vi "Set Output State.vi"(7 "Output Channel":T2, 8 "error in (no error)":errorcluster, 10 "Output State":T1=enum."Enabled", 11 "VISA resource name":refnum<visa-resource-name>) -> (0 "error out":errorcluster, 3 "VISA Refnum out":refnum<visa-resource-name>)   [LabVIEW 2016, in "RP100.lvclass"]
uses:
  RP100.lvclass
  Typedefs/Output Channel--Enum.ctl
  Typedefs/Output State--Enum.ctl
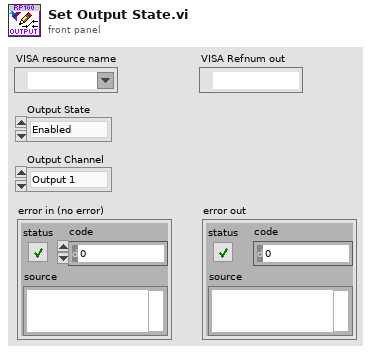
[diagram p1: front panel]
types:
  T1 = typedef "RP100.lvclass/Output State--Enum.ctl" = enum16{"Shorted", "Enabled"}
  T2 = typedef "RP100.lvclass/Output Channel--Enum.ctl" = enum16{"Output 1", "Output 2"}
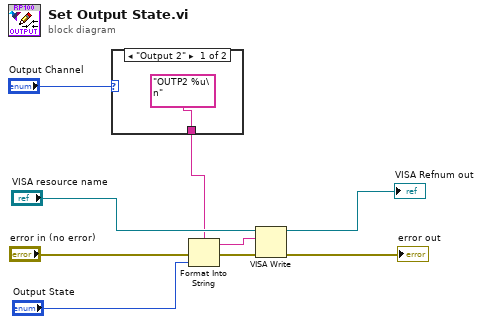
[diagram p0: block diagram]
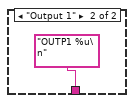
[diagram p2: hidden frame]
diagram:
  n1 = case shown="\"Output 2\"" "Output Channel" {
    tunnel: ["OUTP2 %u\n" ("format string") "OUTP1 %u\n" ("format string")] -> w2
    frame "Output 2" {
    }
    frame "Output 1" {
    }
  }
  n2 = Format Into String(format string=w2, error in="error in (no error)", "Output State") -> (resulting string=w4:string, error out=w3:errorcluster)  [unwired: 1 in]
  n3 = VISA Write(VISA resource name="VISA resource name", write buffer=w4, error in (no error)=w3) -> (VISA resource name out=→"VISA Refnum out":refnum<visa-resource-name>, error out=→"error out":errorcluster)  [unwired: 1 out]
